vi "Read ActorMap.vi"(8 "error in (no error)":errorcluster, 11 "Enqueues Data in":refnum<class "Enqueues Data.lvclass">) -> (0 "error out":errorcluster, 2 "ActorMap.lvclass":refnum<class "ActorMap.lvclass">, 3 "Enqueues Data out":refnum<class "Enqueues Data.lvclass">)   [LabVIEW 2020, in "Enqueues Data.lvclass"]
uses:
  Enqueues Data.lvclass
  C:/Users/yu/Desktop/Pro1/06 Source/Code/Common/ActorMap/ActorMap.lvclass
  Enqueues Data.lvclass/Enqueues Data.ctl
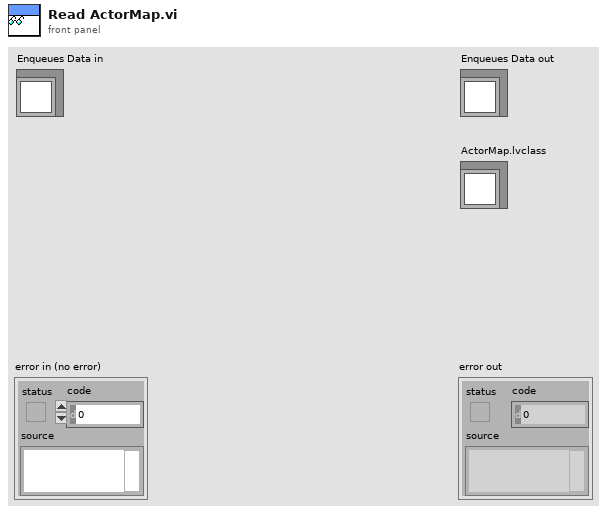
[diagram p1: front panel]
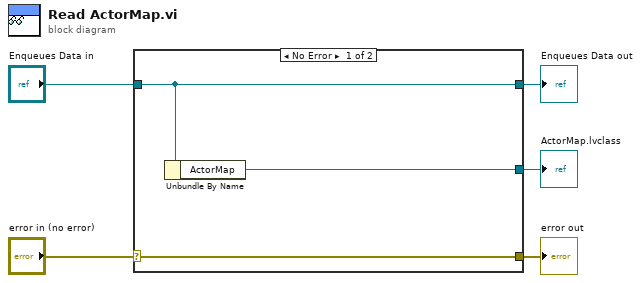
[diagram p0: block diagram]
diagram:
  n1 = case shown="No Error" "error in (no error)" {
    selector: "error in (no error)" -> [w8 w9]
    tunnel: [w8 w9] -> w4
    tunnel: [w7 w10] -> w2
    tunnel: "Enqueues Data in" -> [w7 w10]
    tunnel: [w6 _] -> w1
    frame No Error {
      n2 = Unbundle By Name(w7) -> ("ActorMap"=w6:refnum<class "ActorMap.lvclass">)
    }
    frame Error {
    }
  }
  "error out" <- w4
  "Enqueues Data out" <- w2
  "ActorMap.lvclass" <- w1
